vi "LUTInspectionDlg.vi"   [LabVIEW 2011]
uses:
  GlobalVariables.vi
panel:
  # "LUT Inspection"
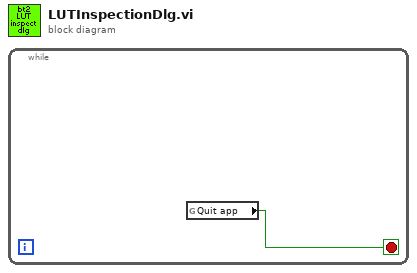
[diagram p0: block diagram]
diagram:
  n1 = while {
    stop <- w1 stop-if-true
    n2 = global read "GlobalVariables.vi" "Quit app"() -> (w1:bool)
  }
